vi "wrapper_DS_read.vi"(1 "String":string) -> (0 "error out":errorcluster)   [LabVIEW 2009]
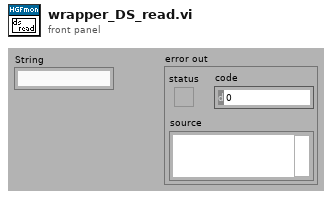
[diagram p1: front panel]
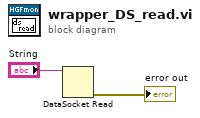
[diagram p0: block diagram]
diagram:
  n1 = DataSocket Read(11:"String") -> (0:→"error out":errorcluster)  [unwired: 1 in, 9 out]
